vi "Write Indexes.vi"(9 "End Out":i32, 10 "Start Out":i32, 11 "(WavIndex_Pointer) In":refnum<class "(WavIndex_Pointer).lvclass">) -> (3 "(WavIndex_Pointer) Out":refnum<class "(WavIndex_Pointer).lvclass">)   [LabVIEW 2016, in "(WavIndex_Pointer).lvclass"]
uses:
  (WavIndex_Pointer).lvclass
  (WavIndex_Pointer).lvclass/(WavIndex_Pointer).ctl
  Index_Pointer/(Index_Pointer).lvclass
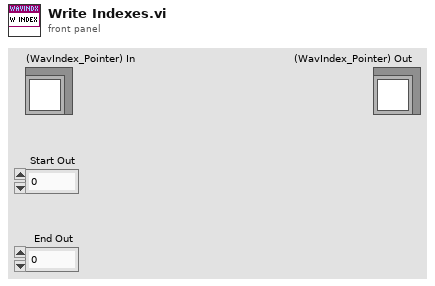
[diagram p1: front panel]
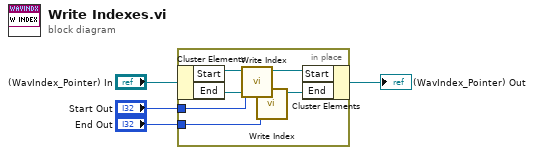
[diagram p0: block diagram]
diagram:
  n1 = in-place {
    in-place-border: "Start Out" -> [w6]
    in-place-border: "End Out" -> [w5]
    n2 = in-place-cluster #1("(WavIndex_Pointer) In") -> ("Start"=w10:refnum<class "(Index_Pointer).lvclass">, "End"=w8:refnum<class "(Index_Pointer).lvclass">)
    n3 = call "Write Index.vi"("Index"=w6, "(Index_Pointer) In"=w10) -> ("(Index_Pointer) Out"=w9:refnum<class "(Index_Pointer).lvclass">)  [unwired: 9 in]
    n4 = call "Write Index.vi"("Index"=w5, "(Index_Pointer) In"=w8) -> ("(Index_Pointer) Out"=w7:refnum<class "(Index_Pointer).lvclass">)  [unwired: 9 in]
    n5 = in-place-cluster #1("Start"=w9, "End"=w7) -> (→"(WavIndex_Pointer) Out":refnum<class "(WavIndex_Pointer).lvclass">)
  }
